vi "Create-reference.vi"(8 "error in (no error)":errorcluster) -> (0 "error out":errorcluster, 2 "Data ref":T1, 3 "PD-Data out":refnum<class "SC-Main.lvclass">)   [LabVIEW 2013, in "SLMControl.lvlib" / "SC-Main.lvclass"]
uses:
  SC-Main.lvclass
  Object-reference.ctl
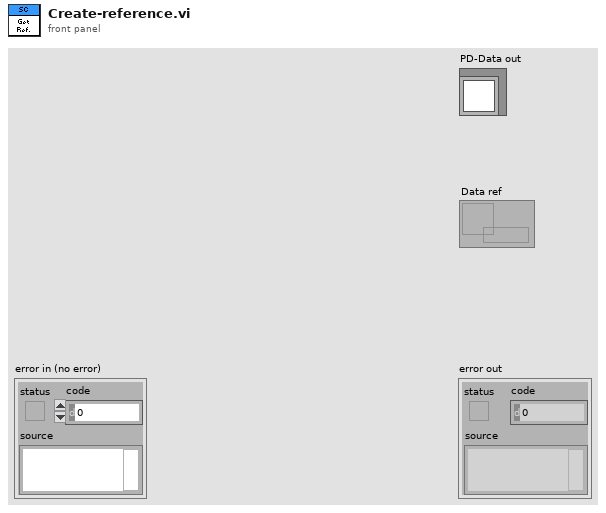
[diagram p1: front panel]
types:
  T1 = typedef "SLMControl.lvlib/SC-Main.lvclass/Object-reference.ctl" = refnum<data-value>
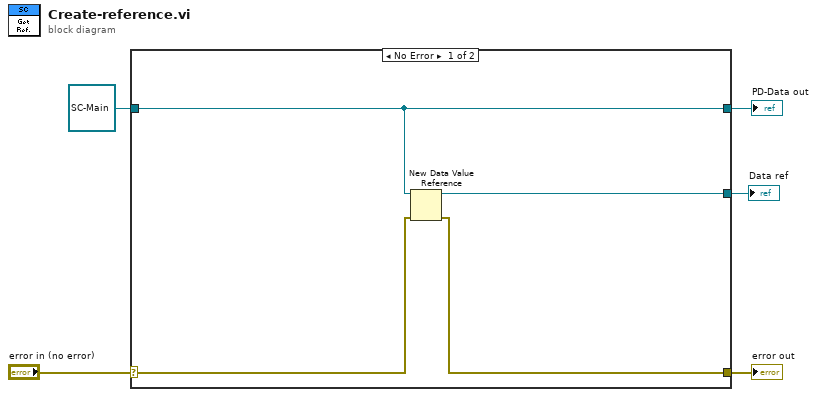
[diagram p0: block diagram]
diagram:
  n1 = case shown="No Error" "error in (no error)" {
    selector: "error in (no error)" -> [w8 w11]
    tunnel: [w7 w11] -> w4
    tunnel: [w9 w10] -> w2
    tunnel: refnum<class "SC-Main.lvclass"> refnum ("PD-Data in") -> [w9 w10]
    tunnel: [w6 _] -> w1
    frame No Error {
      n2 = New Data Value Reference(data value=w9, error in=w8) -> (data value reference=w6:refnum<data-value>, error out=w7:errorcluster)
    }
    frame Error {
    }
  }
  "error out" <- w4
  "PD-Data out" <- w2
  "Data ref" <- w1
